vi "SwissSPAD 1 Format Data.vi"(8 "Error In":errorcluster, 9 "Y Resolution":i32=128, 10 "X Resolution":i32, 11 "Flattened Image":u16[](array[numeric])) -> (0 "Error Out":errorcluster, 3 "Image out":u16[][](array[numeric]))   [LabVIEW 2021, in "SwissSPAD.lvlib"]
uses:
  SwissSPAD.lvlib
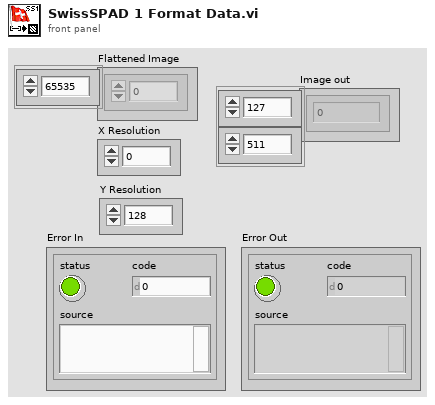
[diagram p1: front panel]
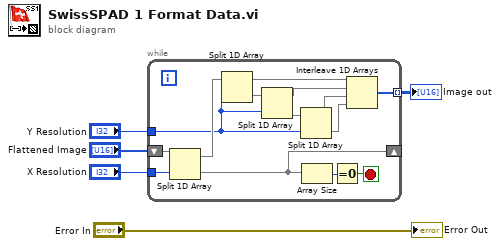
[diagram p0: block diagram]
diagram:
  n1 = while {
    shift-right: [w16] -> _
    shift-left: "Flattened Image" -> [w19]
    tunnel: "X Resolution" -> [w18]
    tunnel: [w17] -> w5 mode=indexing
    tunnel: "Y Resolution" -> [w12]
    stop <- w14 stop-if-true
    n2 = Split 1D Array(array=w19, index=w18) -> (first subarray=w13:u16[], second subarray=w16:u16[])
    n3 = Split 1D Array(array=w13, index=w12) -> (first subarray=w9:u16[], second subarray=w11:u16[])
    n4 = Split 1D Array(array=w11, index=w12) -> (first subarray=w8:u16[], second subarray=w10:u16[])
    n5 = Split 1D Array(array=w10, index=w12) -> (first subarray=w7:u16[], second subarray=w6:u16[])
    n6 = Array Size(array=w16) -> (size(s)=w15:i32)
    n7 = Equal To 0?(x=w15) -> (x = 0?=w14:bool)
    n8 = Interleave 1D Arrays(w9, w8, w7, w6) -> (w17:u16[])
  }
  "Image out" <- w5
  "Error Out" <- "Error In"
